vi "Get Sciscan Scope Zoom.vi"(8 "error in":errorcluster, 11 "GFG Refnum":refnum<vi>) -> (0 "error out":errorcluster, 2 "Current Zoom":dbl=10.0 format="%.2f", 3 "GFG Refnum Out":refnum<vi>)   [LabVIEW 2012, in "Sciscan Scope Daemon.lvlib"]
uses:
  Sciscan Scope Daemon.lvlib
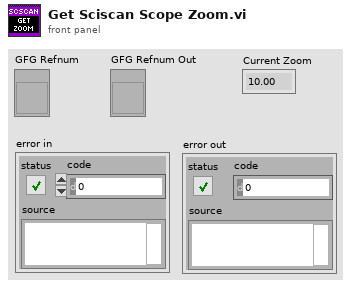
[diagram p1: front panel]
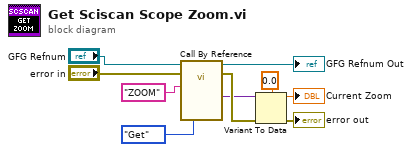
[diagram p0: block diagram]
diagram:
  n1 = call-by-ref "?"(reference="GFG Refnum", error in="error in", "Variable Name in"="ZOOM", "Action"=enum16{"Init", "Set", "Get"}."Get") -> (reference out=→"GFG Refnum Out":refnum<vi>, error out=w6:errorcluster, "Variant Out"=w5:variant)  [unwired: 11 in, 6 out]
  n2 = Variant To Data(error in=w6, type=0.0 ("display every n-th frame"), Variant=w5) -> (data=→"Current Zoom":dbl, error out=→"error out":errorcluster)
